vi "Get Initialize.vi"(8 "error in (no error)":errorcluster, 11 "Abstract Initialize Msg in":refnum<class "Abstract Initialize Msg.lvclass">) -> (0 "error out":errorcluster, 2 "Initialize":bool, 3 "Abstract Initialize Msg out":refnum<class "Abstract Initialize Msg.lvclass">)   [LabVIEW 2013, in "Create Project Model.lvlib" / "Abstract Initialize Msg.lvclass"]
uses:
  Abstract Initialize Msg.lvclass
  Abstract Initialize Msg.lvclass/Abstract Initialize Msg.ctl
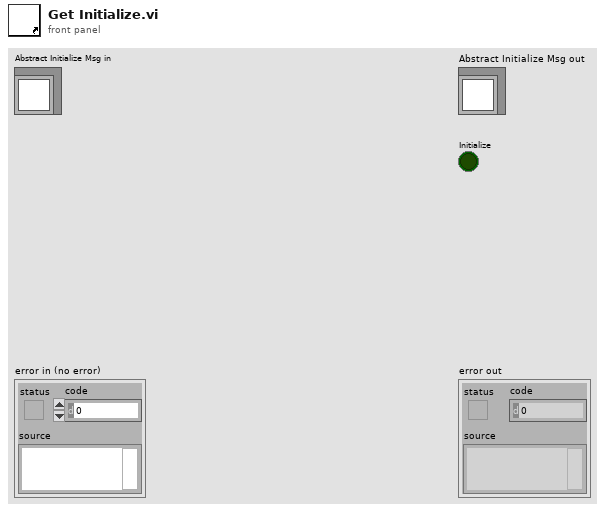
[diagram p1: front panel]
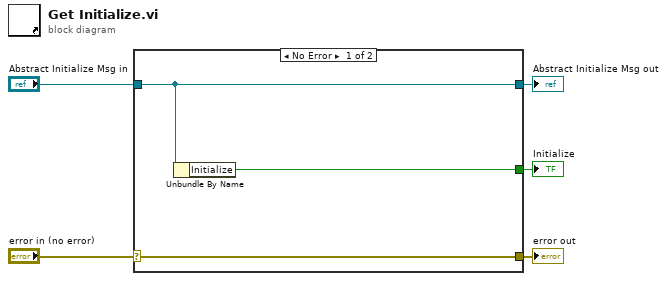
[diagram p0: block diagram]
diagram:
  n1 = case shown="No Error" "error in (no error)" {
    selector: "error in (no error)" -> [w8 w9]
    tunnel: [w8 w9] -> w4
    tunnel: [w7 w10] -> w2
    tunnel: "Abstract Initialize Msg in" -> [w7 w10]
    tunnel: [w6 _] -> w1
    frame No Error {
      n2 = Unbundle By Name(w7) -> ("Initialize"=w6:bool)
    }
    frame Error {
    }
  }
  "error out" <- w4
  "Abstract Initialize Msg out" <- w2
  "Initialize" <- w1
